vi "DSF.Engine.Memory.Cache.Framework.Initialize.vi"(8 "error in (no error)":errorcluster, 10 "Device Ref in":T1=18446744073709551615 format="%.0x", 11 "Framework Cache in":refnum<class "DSF.Engine.Memory.Cache.Framework.lvclass">) -> (0 "error out":errorcluster, 3 "Framework Cache out":refnum<class "DSF.Engine.Memory.Cache.Framework.lvclass">)   [LabVIEW 2016, in "DSF.Engine.lvlib" / "DSF.Engine.Memory.Cache.Framework.lvclass"]
uses:
  DSF.Engine.Memory.Cache.Framework.lvclass
  <vilib>/NI Veristand/Custom Device API/Custom Device Item Ref.ctl
  DSF.Engine.Memory.Cache.Framework.lvclass/DSF.Engine.Memory.Cache.Framework.ctl
  DSF.Engine.Memory.Cache.Plugin.lvclass
  <vilib>/NI Veristand/Custom Device API/Custom Device API.lvlib
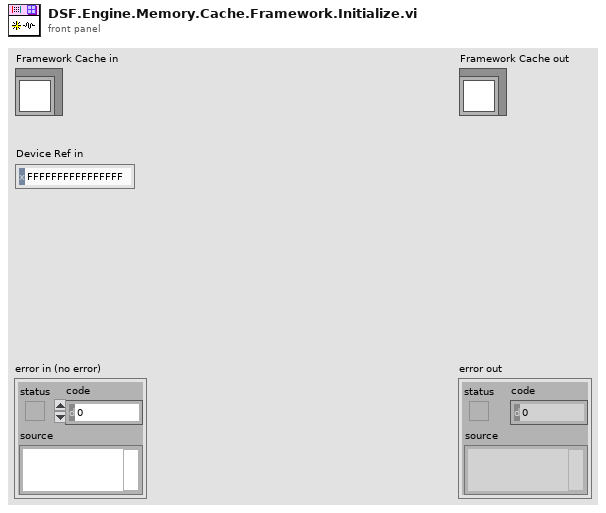
[diagram p1: front panel]
types:
  T1 = typedef "Custom Device API.lvlib/Custom Device Item Ref.ctl" = u64
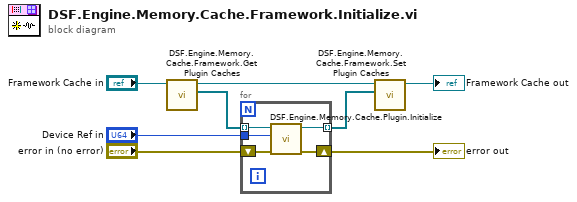
[diagram p0: block diagram]
diagram:
  n1 = call "DSF.Engine.Memory.Cache.Framework.Get Plugin Caches.vi"("Framework Cache in"="Framework Cache in") -> ("Plugin Caches"=w5:refnum<class "DSF.Engine.Memory.Cache.Plugin.lvclass">[], "Framework Cache out"=w7:refnum<class "DSF.Engine.Memory.Cache.Framework.lvclass">)  [unwired: 9 in]
  n2 = for {
    tunnel: [w13] -> w4 mode=indexing
    tunnel: "Device Ref in" -> [w9]
    shift-right: [w12] -> w1
    shift-left: "error in (no error)" -> [w11]
    tunnel: w5 -> [w10] mode=indexing
    n3 = call "DSF.Engine.Memory.Cache.Plugin.Initialize.vi"("error in (no error)"=w11, "Device Ref in"=w9, "Plugin Cache in"=w10) -> ("error out"=w12:errorcluster, "Plugin Cache out"=w13:refnum<class "DSF.Engine.Memory.Cache.Plugin.lvclass">)  [unwired: 7 in]
  }
  "error out" <- w1
  n4 = call "DSF.Engine.Memory.Cache.Framework.Set Plugin Caches.vi"("Plugin Caches"=w4, "Framework Cache in"=w7) -> ("Framework Cache out"=→"Framework Cache out":refnum<class "DSF.Engine.Memory.Cache.Framework.lvclass">)  [unwired: 9 in]
